vi "GetFrontPanel.vi"(8 "Error In":errorcluster, 11 "object in":refnum<class "Mockup_UserManager.lvclass">) -> (0 "Error Out":errorcluster, 2 "FrontPanel":refnum<class "FrontPanelControl.lvclass">, 3 "object out":refnum<class "Mockup_UserManager.lvclass">)   [LabVIEW 2021, in "Mockup_UserManager.lvclass"]
uses:
  Mockup_UserManager.lvclass
  .Externals/Library_UserInterface_FrontPanelControl/FrontPanelControl/FrontPanelControl.lvclass
  Mockup_UserManager.lvclass/Mockup_UserManager.ctl
panel:
  in  "Items":u16(ring)
  in  "AuthorizationLevels":i32(listbox)
  in  "Save 4":bool
  in  "Save 3":bool
  in  "Save 2":bool
  in  "Functions":i32(listbox)
  in  "Save 7":bool
  in  "Save 6":bool
  in  "Save 5":bool
  in  "Users":i32(listbox)
  in  "Save 10":bool
  in  "Save 9":bool
  in  "Save 8":bool
  in  "Save":bool
  in  "Cancel":bool
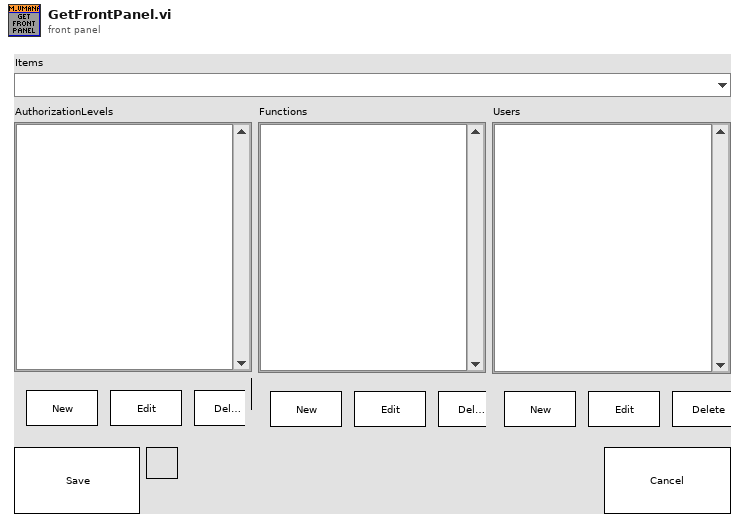
[diagram p1: front panel]
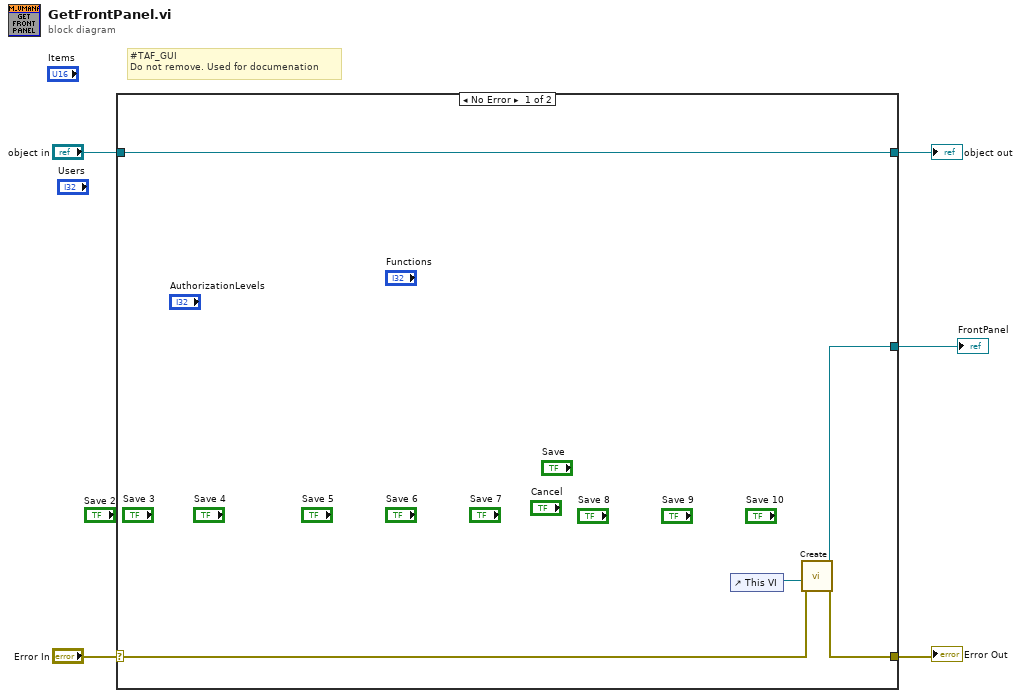
[diagram p0: block diagram]
diagram:
  # "#TAF_GUI\nDo not remove. Used for documenation"
  n1 = case shown="No Error" "Error In" {
    selector: "Error In" -> [w8 w12]
    tunnel: [w7 w12] -> w4
    tunnel: [w10 w11] -> w2
    tunnel: "object in" -> [w10 w11]
    tunnel: [w6 _] -> w1
    frame No Error {
      n2 = control-ref of="This VI"() -> (w9:refnum<vi>)
      n3 = call "Create.vi"("ErrorIn"=w8, "VIRef"=w9) -> ("ErrorOut"=w7:errorcluster, "ObjectOut"=w6:refnum<class "FrontPanelControl.lvclass">)  [unwired: 8 in]
    }
    frame Error {
    }
  }
  "Error Out" <- w4
  "object out" <- w2
  "FrontPanel" <- w1
